vi "Bind Terminal Enabled State.vi"(4 "FALSE State (Disabled and Grayed Out)":T1(ring)=enum."Disabled and Grayed Out", 6 "TRUE State (Enabled)":T1(ring), 7 "Initial State (T)":bool=TRUE, 8 "error in (no error)":errorcluster, 9 "Datum Name (\"\"=Use Control Label)":string, 10 "Ctl Refnum":refnum<vi>, 11 "IViewable in":refnum<class "IViewable.lvclass">) -> (0 "error out":errorcluster, 3 "IViewable out":refnum<class "IViewable.lvclass">)   [LabVIEW 2020, in "IViewable.lvlib" / "IViewable.lvclass"]
doc: "Bind the enabled state of a control terminal (control or indicator) to a published Boolean or Numeric datum. Specify the logical relationship between datum vale and terminal state by wiring the optional input terminals.\n\nDefault for Boolean:\nPublished TRUE = Enabled\nPublished FALSE = Disabled and Grayed Out\n\nDefault for Numeric:\nPublised value greater than 0 = Enabled\nPublished value NOT greater than 0 = Disabled and Grayed Out"
uses:
  IViewable.lvclass
  IViewable.lvclass/IViewable.ctl
  mva-core/Source/IMediator/SubscriptionRequest/SubscriptionRequest.lvclass
  mva-core/Source/IObserver/IObserver Messages/Subscribe Msg/Subscribe Msg.lvclass
  <vilib>/ActorFramework/Actor/Actor.lvclass
  mva-core/Source/IMediator/ISubscriptionPolicy/ISubscriptionPolicy.lvclass
  mva-core/Source/SubscriptionPolicy/ValueChangeSubscription/ValueChangeSubscription.lvclass
  <vilib>/Utility/Data Type/NI_Data Type.lvlib
  composed-transport/Source/Concrete/TerminalEnabledStateBinding/TerminalEnabledStateBinding.lvclass
  C:/Program Files/National Instruments/LabVIEW 2020/vi.lib/ActorFramework/Actor/Actor.lvclass
panel:
  in  "Datum Type (Boolean)":variant
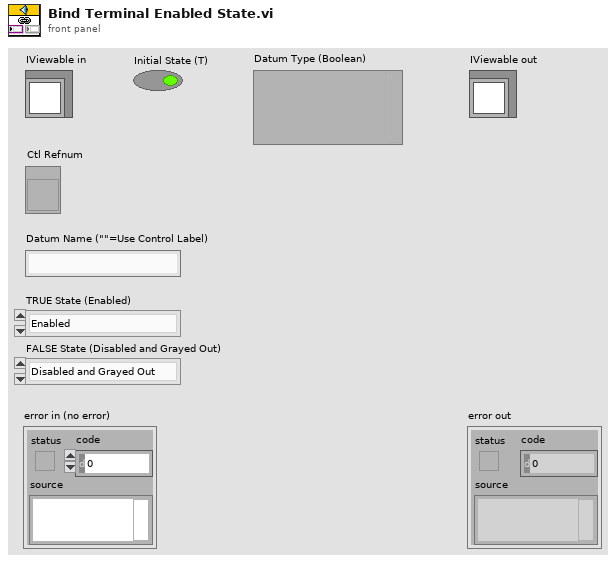
[diagram p1: front panel]
types:
  T1 = enum8{"Enabled", "Disabled", "Disabled and Grayed Out"}
  T2 = typedef "NI_Data Type.lvlib/Data Type.ctl" = enum8{"Invalid Type", "Void", "I8", "I16", "I32", "I64", "U8", "U16", "U32", "U64", "Single Float", "Double Float", "Extended Float", "Single Complex", "Double Complex", "Extended Complex", "Enum U8", "Enum U16", "Enum U32", "Enum U64", "Single Float With Unit", "Double Float With Unit", "Extended Float With Unit", "Single Complex with Unit", "Double Complex with Unit", "Extended Complex with Unit", "Boolean", "String", "Path", "Picture", "Tag", "Array", "Cluster", "Variant", "LV Variant", "Waveform", "Timestamp", "Digital Waveform", "Digital Data", "ExpressData", "Refnum", "External Data", "VI", "Poly VI", "LabVIEW Class Instance", "Fixed Point", "Set Collection", "Map Collection"}
  T3 = typedef "IMediator.lvlib/ISubscriptionPolicy.lvclass/ISubscriptionPolicy Reference.ctl" = refnum<data-value>
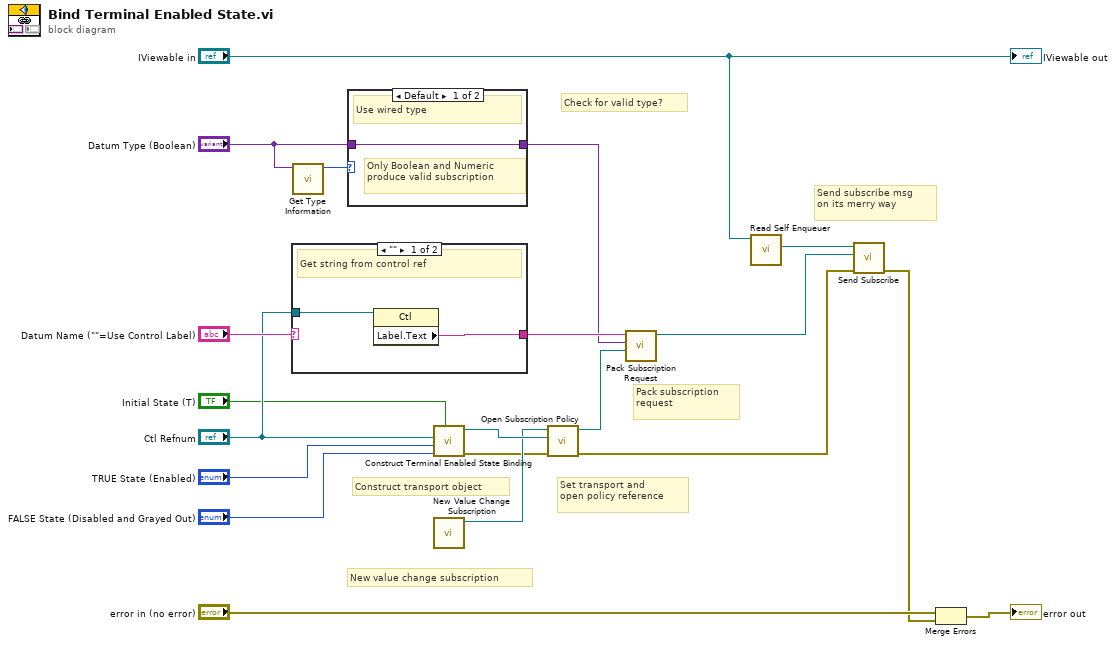
[diagram p0: block diagram]
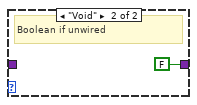
[diagram p2: hidden frame]
diagram:
  # "Check for valid type?"
  # "New value change subscription"
  # "Set transport and\nopen policy reference"
  # "Send subscribe msg\non its merry way"
  # "Pack subscription\nrequest"
  # "Construct transport object"
  n1 = case shown="\"\"" "Datum Name (\"\"=Use Control Label)" {
    selector: "Datum Name (\"\"=Use Control Label)" -> [_ w23]
    tunnel: [w21 w23] -> w13
    tunnel: "Ctl Refnum" -> [w22 _]
    frame "" {
      # "Get string from control ref"
      n2 = property class="Ctl"(reference=w22) -> ("Label.Text"=w21:string)  [unwired: 1 in, 2 out]
    }
    frame Default {
      # "Use string wired to input terminal"
    }
  }
  n3 = call <vilib>:"Get Type Information.vi"("variant"="Datum Type (Boolean)") -> ("type"=w5:T2)  [unwired: 6 in, 4 out]
  n4 = case shown="Default" w5 {
    tunnel: [w24 FALSE] -> w4
    tunnel: "Datum Type (Boolean)" -> [w24 _]
    frame Default {
      # "Only Boolean and Numeric\nproduce valid subscription"
      # "Use wired type"
    }
    frame "Void" {
      # "Boolean if unwired"
    }
  }
  n5 = call "Construct Terminal Enabled State Binding.vi"("Initial State (T)"="Initial State (T)", "FALSE State (Disabled and Grayed Out)"="FALSE State (Disabled and Grayed Out)", "TRUE State (Enabled)"="TRUE State (Enabled)", "Control"="Ctl Refnum") -> ("error out"=w6:errorcluster, "TerminalEnabledStateBinding"=w11:refnum<class "TerminalEnabledStateBinding.lvclass">)  [unwired: 6 in]
  n6 = call "New Value Change Subscription.vi"() -> ("ValueChangeSubscription Out"=w10:refnum<class "ValueChangeSubscription.lvclass">)  [unwired: 11 in]
  n7 = call "Open Subscription Policy.vi"("error in (no error)"=w6, "Transport"=w11, "SubscriptionPolicy"=w10) -> ("error out"=w1:errorcluster, "Subscription Policy"=w2:T3)  [unwired: 7 in]
  n8 = call "Pack Subscription Request.vi"("Subscription Policy"=w2, "Type"=w4, "Datum Name"=w13) -> ("SubscriptionRequest"=w17:refnum<class "SubscriptionRequest.lvclass">)  [unwired: 7 in, 1 out]
  n9 = call <vilib>:"Read Self Enqueuer.vi"("Actor"="IViewable in") -> ("Self Enqueuer"=w18:refnum<class "Message Enqueuer.lvclass">)  [unwired: 10 in]
  n10 = call "Send Subscribe.vi"("error in (no error)"=w1, "SubscriptionRequest"=w17, "Message Enqueuer"=w18) -> ("error out"=w15:errorcluster)  [unwired: 7 in, 1 out]
  n11 = Merge Errors("error in (no error)", w15) -> (→"error out":errorcluster)
  "IViewable out" <- "IViewable in"
